vi "Render Section Children.vi"(8 "Error In":errorcluster, 10 "Section":refnum<class "Section.lvclass">, 11 "Renderer In":refnum<class "Renderer.lvclass">) -> (0 "Error Out":errorcluster, 2 "Output":string, 3 "Renderer Out":refnum<class "Renderer.lvclass">)   [LabVIEW 2018, in "Toolkit.lvlib" / "Renderer.lvclass"]
uses:
  Renderer.lvclass
  Nodes/Section/Section.lvclass
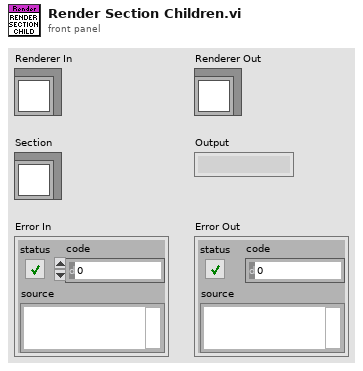
[diagram p1: front panel]
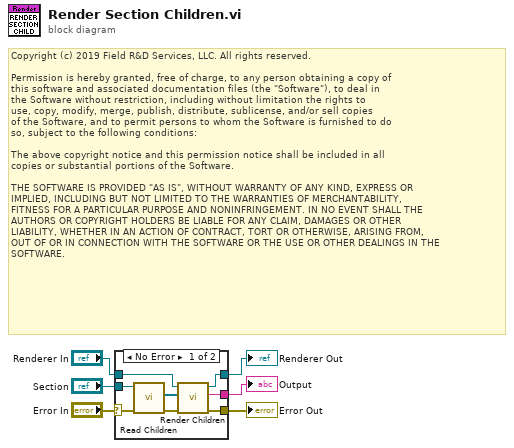
[diagram p0: block diagram]
diagram:
  # "Copyright (c) 2019 Field R&D Services, LLC. All rights reserved.\n\nPermission is hereby granted, free of charge, to any person obtaining a copy of\nthis software and associated documentation files (the \"Software\"), to deal in\nthe Software without restriction, including without limitation the rights to\nuse, copy, modify, merge, publish, distribute, sublicense, and/or sell copies\nof the Software, and to permit persons to whom the Software is furnished to do\nso, subject to the following conditions:\n\nThe above copyright notice and this permission notice shall be included in all\ncopies or substantial portions of the Software.\n\nTHE SOFTWARE IS PROVIDED \"AS IS\", WITHOUT WARRANTY OF ANY KIND, EXPRESS OR\nIMPLIED, INCLUDING BUT NOT LIMITED TO THE WARRANTIES OF MERCHANTABILITY,\nFITNESS FOR A PARTICULAR PURPOSE AND NONINFRINGEMENT. IN NO EVENT SHALL THE\nAUTHORS OR COPYRIGHT HOLDERS BE LIABLE FOR ANY CLAIM, DAMAGES OR OTHER\nLIABILITY, WHETHER IN AN ACTION OF CONTRACT, TORT OR OTHERWISE, ARISING FROM,\nOUT OF OR IN CONNECTION WITH THE SOFTWARE OR THE USE OR OTHER DEALINGS IN THE\nSOFTWARE."
  n1 = case shown="No Error" "Error In" {
    selector: "Error In" -> [w13 w16]
    tunnel: [w10 w16] -> w6
    tunnel: "Section" -> [w14 _]
    tunnel: [w11 w15] -> w1
    tunnel: [w8 _] -> w3
    tunnel: "Renderer In" -> [w7 w15]
    frame No Error {
      n2 = call-dynamic "Read Children.vi"("Error In"=w13, "Non-Terminal In"=w14) -> ("Error Out"=w9:errorcluster, "Children"=w12:refnum<class "Node.lvclass">[])  [unwired: 7 in, 1 out]
      n3 = call "Render Children.vi"("Error In"=w9, "Children"=w12, "Renderer In"=w7) -> ("Error Out"=w10:errorcluster, "Output"=w8:string, "Renderer Out"=w11:refnum<class "Renderer.lvclass">)  [unwired: 6 in]
    }
    frame Error {
    }
  }
  "Output" <- w3
  "Error Out" <- w6
  "Renderer Out" <- w1
